vi "Configure PRACH Frequency Offset.vi"(7 "Frequency Offset (0)":i32, 8 "error in (no error)":errorcluster, 9 "Frequency Offset Auto (On)":bool=TRUE, 10 "Instance (1)":T1=1, 11 "VISA resource name":refnum<visa-resource-name>) -> (0 "error out":errorcluster, 3 "VISA resource name out":refnum<visa-resource-name>)   [LabVIEW 2020, in "Rohde&Schwarz CMWXP NR FR1 Measurement.lvlib"]
doc: "Enables or disables automatic detection of the PRACH frequency offset. Specifies the PRACH frequency offset if automatic detection is disabled.\n\nAttributes:\nRSCMWXPNRFR1M_ATTR_PRACH_FREQUENCY_OFFSET_ENABLED\nRSCMWXPNRFR1M_ATTR_PRACH_FREQUENCY_OFFSET\n\nRemote-control commands:\nCONFigure:NRSub:MEAS<i>:PRACh:PFOFfset:AUTO\nCONFigure:NRSub:MEAS<i>:PRACh:PFOFfset"
uses:
  <instrlib>/Rohde&Schwarz CMWXP NR FR1 Measurement/Rohde&Schwarz CMWXP NR FR1 Measurement.lvlib
  <instrlib>/Rohde&Schwarz CMWXP NR FR1 Measurement/Private/_Instance.ctl
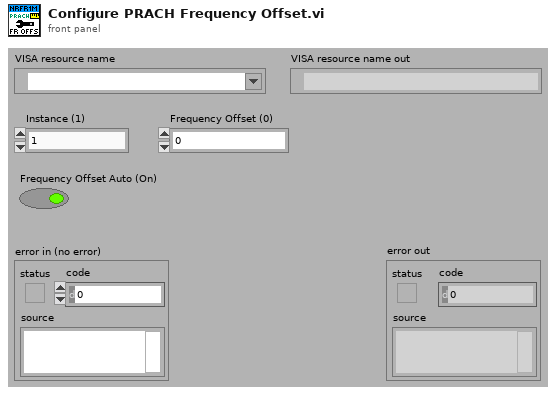
[diagram p1: front panel]
types:
  T1 = typedef "Rohde&Schwarz CMWXP NR FR1 Measurement.lvlib/_Instance.ctl" = i32
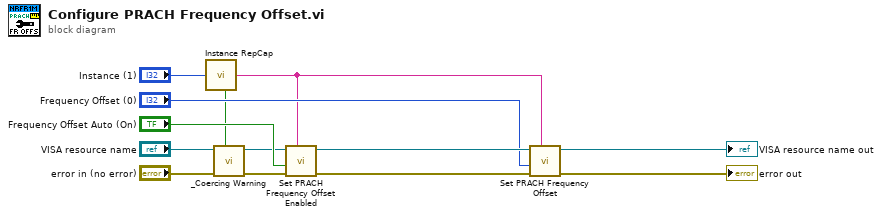
[diagram p0: block diagram]
diagram:
  n1 = call <instrlib>:"Instance RepCap.vi"("Instance In"="Instance (1)") -> ("In Range?"=w2:bool, "RepCap Identifier Out"=w1:string)  [unwired: 1 in]
  n2 = call <instrlib>:"_Coercing Warning.vi"("In Range?"=w2, "error in (no error)"="error in (no error)", "VISA resource name"="VISA resource name") -> ("error out"=w5:errorcluster, "VISA resource name out"=w4:refnum<visa-resource-name>)  [unwired: 7 in]
  n3 = call "Set PRACH Frequency Offset Enabled"("Repeated Capabilities"=w1, "error in (no error)"=w5, "PRACH Frequency Offset Enabled (OFF)"="Frequency Offset Auto (On)", "instrument handle"=w4) -> ("error out"=w9:errorcluster, "instrument handle out"=w10:refnum<visa-resource-name>)  [unwired: 6 in]
  n4 = call "Set PRACH Frequency Offset"("Repeated Capabilities"=w1, "error in (no error)"=w9, "PRACH Frequency Offset (0)"="Frequency Offset (0)", "instrument handle"=w10) -> ("error out"=→"error out":errorcluster, "instrument handle out"=→"VISA resource name out":refnum<visa-resource-name>)  [unwired: 6 in]
